vi "SCRIPT CREATE DB.vi"(8 "error in":errorcluster, 10 "class":refnum<class "_ISerializable.lvclass">) -> (0 "error out":errorcluster, 1 "drop-create script":string, 2 "create script":string)   [LabVIEW 2018, in "ORM Scripter.lvclass"]
uses:
  ORM Scripter.lvclass
  _Serializable Base Object/_ISerializable.lvclass
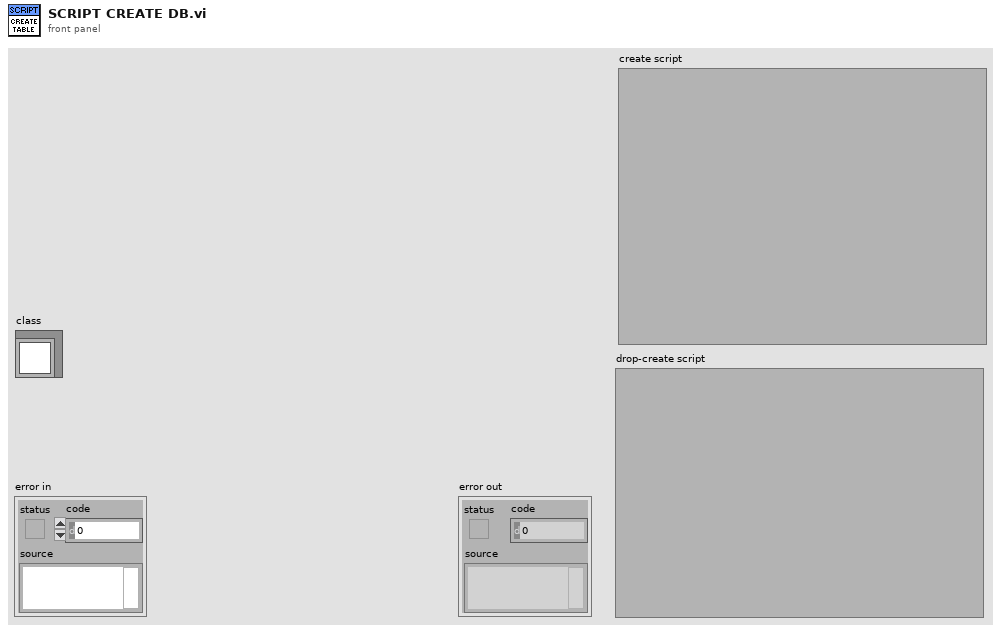
[diagram p1: front panel]
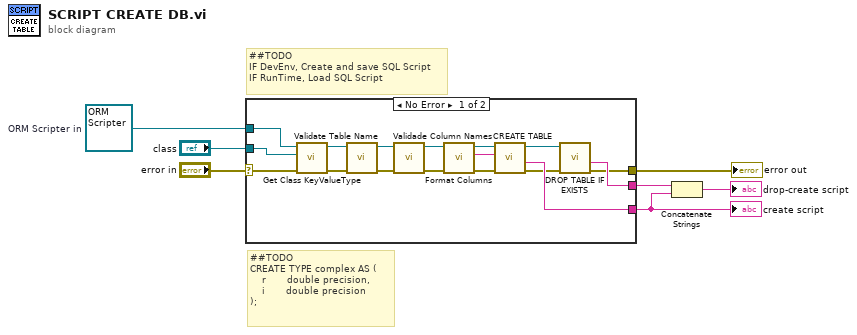
[diagram p0: block diagram]
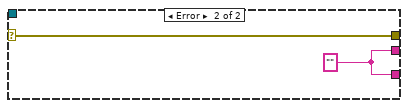
[diagram p2: hidden frame]
diagram:
  w5 = refnum<class "ORM Scripter.lvclass"> refnum  # ORM Scripter in
  # "##TODO\nCREATE TYPE complex AS (\n    r       double precision,\n    i       double precision\n);"
  # "##TODO\nIF DevEnv, Create and save SQL Script\nIF RunTime, Load SQL Script"
  n1 = case shown="No Error" "error in" {
    selector: "error in" -> [w21 w26]
    tunnel: [w9 w26] -> w6
    tunnel: w5 -> [w24 _]
    tunnel: "class" -> [w22 _]
    tunnel: [w11 w25] -> w2
    tunnel: [w17 w25] -> w3
    frame No Error {
      n2 = call "Get Class KeyValueType.vi"("error in (no error)"=w21, "class"=w22, "ORM Scripter in"=w24) -> ("error out"=w20:errorcluster, "ORM Scripter out"=w23:refnum<class "ORM Scripter.lvclass">)  [unwired: 7 in]
      n3 = call "Validate Table Name.vi"("error in (no error)"=w20, "ORM Scripter in"=w23) -> ("error out"=w14:errorcluster, "ORM Scripter out"=w15:refnum<class "ORM Scripter.lvclass">)  [unwired: 8 in]
      n4 = call "Validade Column Names.vi"("error in (no error)"=w14, "ORM Scripter in"=w15) -> ("error out"=w12:errorcluster, "ORM Scripter out"=w13:refnum<class "ORM Scripter.lvclass">)  [unwired: 8 in]
      n5 = call "Format Columns.vi"("error in (no error)"=w12, "ORM Scripter in"=w13) -> ("error out"=w18:errorcluster, "String"=w8:string, "ORM Scripter out"=w19:refnum<class "ORM Scripter.lvclass">)  [unwired: 7 in]
      n6 = call "CREATE TABLE.vi"("error in"=w18, "cols & types"=w8, "ORM Scripter in"=w19) -> ("error out"=w10:errorcluster, "create script"=w11:string, "ORM Scripter out"=w16:refnum<class "ORM Scripter.lvclass">)  [unwired: 6 in]
      n7 = call "DROP TABLE IF EXISTS.vi"("error in (no error)"=w10, "ORM Scripter in"=w16) -> ("error out"=w9:errorcluster, "Drop if exists"=w17:string)  [unwired: 7 in, 1 out]
    }
    frame Error {
      w25 = ""
    }
  }
  "error out" <- w6
  "create script" <- w2
  n8 = Concatenate Strings(w3, w2) -> (→"drop-create script":string)
